vi "Txt to clean Array (Dashboard).vi"(3 "error in":errorcluster, 4 "Overide":bool, 5 "Variables":string, 6 "file path":path=path "C:/Users/usr/Desktop/FRC/2014 code/Robot Constants 2-3-14.txt") -> (0 "error out":errorcluster, 1 "Variable Names":string[](array[string]), 2 "Array of Numbers":dbl[](array[numeric]))   [LabVIEW 2013]
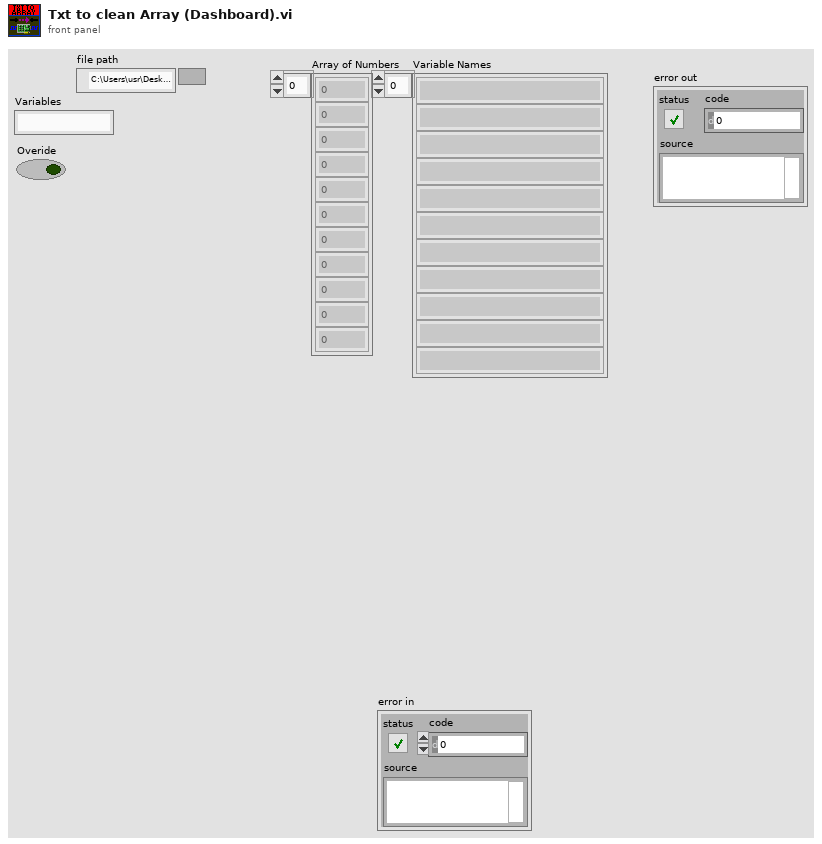
[diagram p1: front panel]
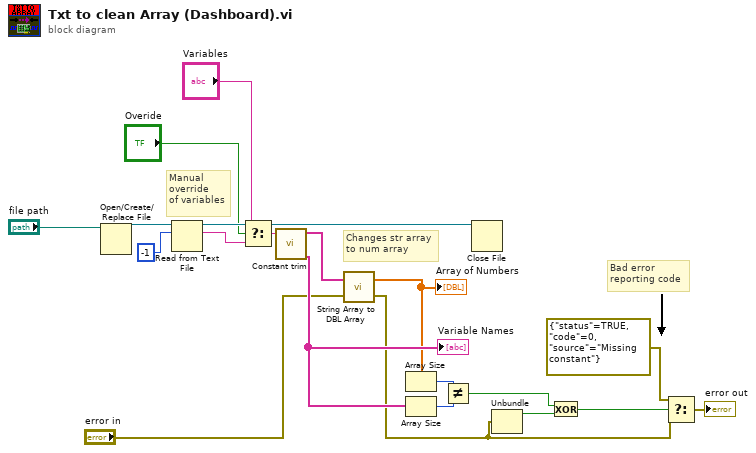
[diagram p0: block diagram]
diagram:
  # "Bad error \nreporting code"
  # "Manual\noverride\nof variables"
  # "Changes str array\nto num array"
  n1 = Open/Create/Replace File(file path (use dialog)="file path") -> (refnum out=w19:refnum<file>)  [unwired: 5 in, 2 out]
  n2 = Read from Text File(file (use dialog)=w19, count=-1) -> (refnum out=w18:refnum<file>, text=w3:string)  [unwired: 2 in, 2 out]
  n3 = Select(t="Variables", s="Overide", f=w3) -> (s? t:f=w4:string)
  n4 = call "Constant trim.vi"("String"=w4) -> ("Array of Names"=w16:string[], "Array of Numbers"=w11:string[])  [unwired: 9 in]
  "Variable Names" <- w16
  n5 = call "String Array to DBL Array.vi"("error in"="error in", "Array of Numbers"=w11) -> ("Error out"=w8:errorcluster, "Array of Numbers"=w10:dbl[])
  "Array of Numbers" <- w10
  n6 = Array Size(array=w10) -> (size(s)=w14:i32)
  n7 = Array Size(array=w16) -> (size(s)=w15:i32)
  n8 = Not Equal?(x=w14, y=w15) -> (x != y?=w7:bool)
  n9 = Close File(refnum=w18) -> ()  [unwired: 1 in, 2 out]
  n10 = Unbundle(w8) -> ("status"=w5:bool)  [unwired: 2 out]
  n11 = Exclusive Or(1:w5, 2:w7) -> (0:w6:bool)
  n12 = Select(t=errorcluster {"status"=TRUE, "code"=0, "source"="Missing constant"} ("error in"), s=w6, f=w8) -> (s? t:f=→"error out":errorcluster)
